vi "Initialize XML.vi"   [LabVIEW 2016, in "SLL File IO.lvlib"]
uses:
  SLL File IO.lvlib
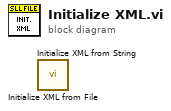
[diagram p0: block diagram]
diagram:
  n1 = call "Initialize XML from File.vi"() -> ()  [unwired: 10 in, 2 out]
  n2 = call "Initialize XML from String.vi"() -> ()  [unwired: 10 in, 2 out]
